vi "Handle Transceiver Error.vi"(8 "error in (no error)":errorcluster, 10 "transceiver error":errorcluster, 11 "Framework in":refnum<class "Framework.lvclass">) -> (0 "error out":errorcluster, 3 "Framework out":refnum<class "Framework.lvclass">)   [LabVIEW 2017, in "DSF Core.lvlib" / "Framework.lvclass"]
uses:
  Framework.lvclass
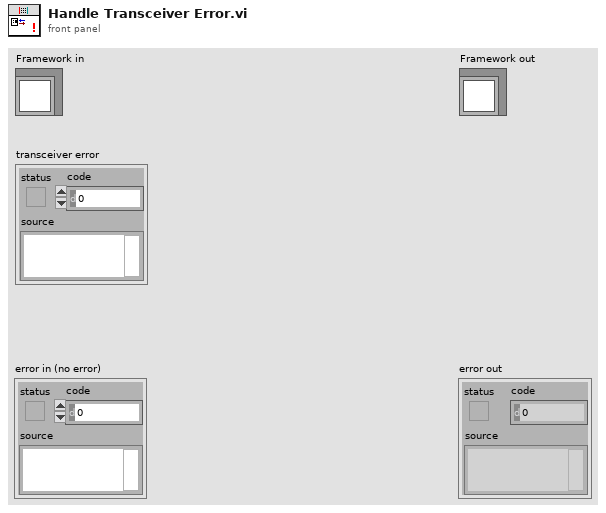
[diagram p1: front panel]
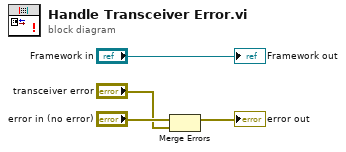
[diagram p0: block diagram]
diagram:
  n1 = Merge Errors("error in (no error)", "transceiver error") -> (→"error out":errorcluster)
  "Framework out" <- "Framework in"
